vi "Untitled 2.vi"() -> ()   [LabVIEW 2017]
uses:
  <vilib>/sound2/lvsound2.llb/Sampling Mode.ctl
  <vilib>/sound2/lvsound2.llb/Sound Data Format.ctl
  Control 1.ctl
  <vilib>/sound2/lvsound2.llb/Sound Input Read (DBL).vi
panel:
  out "error out":errorcluster
  in  "?":bool
  out "Enum":T1
  in  "device ID":u32
  in  "sound format":T2={"sample rate (S/s)"=22050.0, "number of channels"=2, "bits per sample"=16}
  in  "sample mode":T3=1 items=["Finite Samples", "Continuous Samples"]
  in  "number of samples/ch 2":i32=100000
  out "Time Signal":waveform(dbl)[](graph)
  in  "?":bool
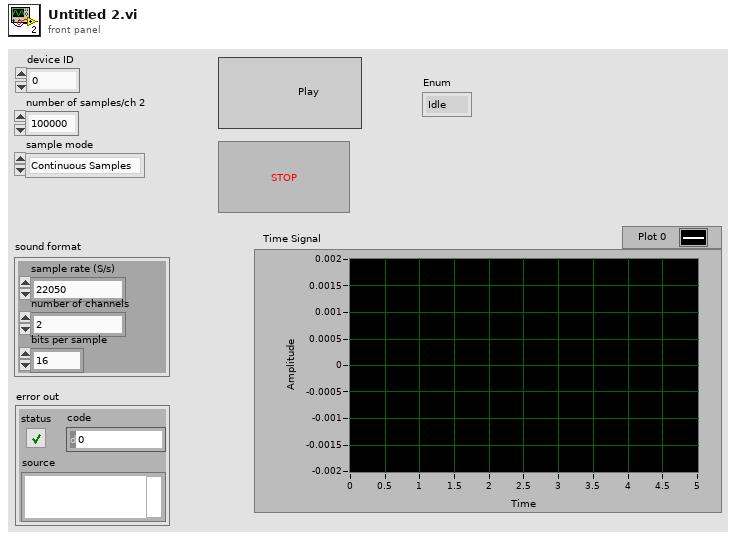
[diagram p1: front panel]
types:
  T1 = typedef "Control 1.ctl" = enum16{"Idle", "Initialization", "Aquisition", "End"}
  T2 = typedef "Sound Data Format.ctl" = cluster{"sample rate (S/s)":dbl, "number of channels":i32, "bits per sample":i32}
  T3 = typedef "Sampling Mode.ctl" = i32
  T4 = typedef "Sound Input Task ID.ctl" = u32
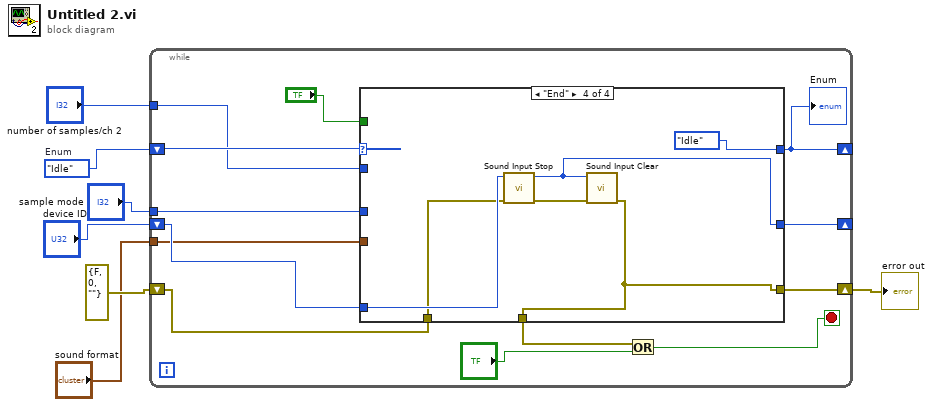
[diagram p0: block diagram]
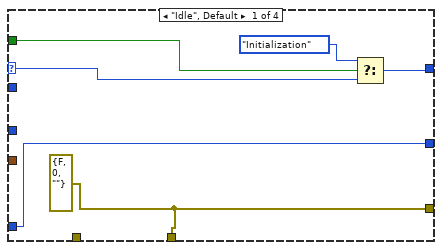
[diagram p2: hidden frame]
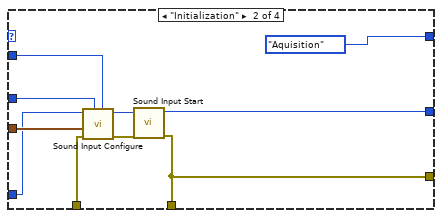
[diagram p3: hidden frame]
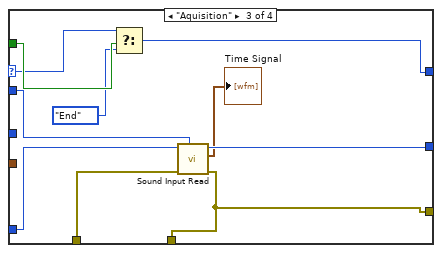
[diagram p4: hidden frame]
diagram:
  w5 = Control_1."Idle"  # Enum
  n1 = while {
    shift-right: [w16] -> _
    shift-left: w5 -> [w11]
    shift-right: [w14] -> w1
    shift-left: errorcluster {"status"=FALSE, "code"=0, "source"=""} ("error in (no error)") -> [w17]
    shift-right: [w13] -> _
    shift-left: "device ID" -> [w12]
    tunnel: "sample mode" -> [w10]
    tunnel: "sound format" -> [w9]
    tunnel: "number of samples/ch 2" -> [w8]
    stop <- w18 stop-if-true
    n2 = case shown="\"End\"" w11 {
      selector: w11 -> [w23 _ w37 _]
      tunnel: [w25 Control_1."Aquisition" ("Enum") w41 Control_1."Idle" ("Enum")] -> w16
      tunnel: "?" -> [w26 _ w43 _]
      tunnel: [w22 w36 w45 w50] -> w19
      tunnel: [w22 w36 w45 w50] -> w14
      tunnel: [w21 w35 w46 w51] -> w13
      tunnel: w17 -> [_ w31 w40 w47]
      tunnel: w9 -> [_ w30 _ _]
      tunnel: w10 -> [_ w29 _ _]
      tunnel: w8 -> [_ w28 w38 _]
      tunnel: w12 -> [w21 w27 w39 w48]
      frame "Idle", Default {
        w22 = errorcluster {"status"=FALSE, "code"=0, "source"=""} ("error out")
        n3 = Select(t=Control_1."Initialization" ("Enum"), s=w26, f=w23) -> (s? t:f=w25:T1)
      }
      frame "Initialization" {
        n4 = call <vilib>:"Sound Input Configure.vi"("number of samples/ch"=w28, "sample mode"=w29, "error in (no error)"=w31, "sound format"=w30, "device ID"=w27) -> ("error out"=w32:errorcluster, "task ID"=w33:T4)  [unwired: 5 in]
        n5 = call <vilib>:"Sound Input Start.vi"("error in (no error)"=w32, "task ID"=w33) -> ("error out"=w36:errorcluster, "task ID out"=w35:T4)  [unwired: 8 in]
      }
      frame "Aquisition" {
        n6 = Select(t=w37, s=w43, f=Control_1."End" ("Enum")) -> (s? t:f=w41:T1)
        n7 = call-poly <vilib>:"Sound Input Read.vi"("number of samples/ch"=w38, "error in (no error)"=w40, "task ID"=w39) -> ("error out"=w45:errorcluster, "data"=→"Time Signal":waveform(dbl)[], "task ID out"=w46:T4)  [unwired: 6 in]
      }
      frame "End" {
        n8 = call <vilib>:"Sound Input Stop.vi"("error in (no error)"=w47, "task ID"=w48) -> ("error out"=w52:errorcluster, "task ID out"=w51:T4)  [unwired: 8 in]
        n9 = call <vilib>:"Sound Input Clear.vi"("error in (no error)"=w52, "task ID"=w51) -> ("error out"=w50:errorcluster)  [unwired: 9 in]
      }
    }
    "Enum" <- w16
    n10 = Or(x=w19, y="?") -> (x .or. y?=w18:bool)
  }
  "error out" <- w1
